vi "construct.vi"(8 "error in (no error)":errorcluster, 9 "configuration name":string, 10 "load config file?":bool=TRUE, 11 "StimulatorDL090824Gate in":refnum<class "StimulatorDL090824Gate.lvclass">) -> (0 "error out":errorcluster, 3 "StimulatorDL090824Gate out":refnum<class "StimulatorDL090824Gate.lvclass">)   [LabVIEW 2010, in "StimulatorDL090824Gate.lvclass"]
uses:
  StimulatorDL090824Gate.lvclass
  StimulatorDL090724Scaffold/StimulatorDL090724Scaffold/Stimulator090724Scaffold.lvclass
  StimulatorDL090824Gate.lvclass/StimulatorDL090824Gate.ctl
  common/classes/ErrorController/ErrorController/class_data.vi
  common/classes/ErrorController/ErrorController/ErrorController.lvclass
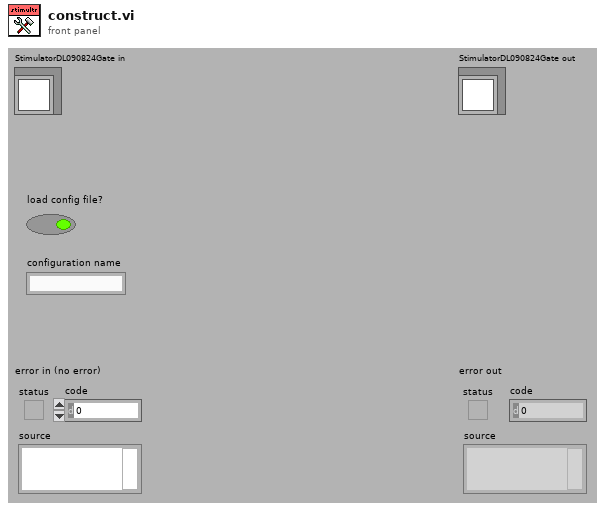
[diagram p1: front panel]
types:
  T1 = typedef "plugin_specification.ctl" = cluster{"class path":string, "configuration":string, "label":string, "settings name":string}
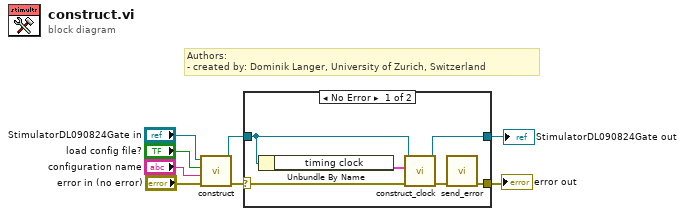
[diagram p0: block diagram]
diagram:
  # "Authors: \n- created by: Dominik Langer, University of Zurich, Switzerland"
  n1 = call-parent "construct.vi"("error in (no error)"="error in (no error)", "configuration name"="configuration name", "load config file?"="load config file?", "GenericPlugin in"="StimulatorDL090824Gate in") -> ("error out"=w4:errorcluster, "GenericPlugin out"=w3:refnum<class "StimulatorDL090824Gate.lvclass">)  [unwired: 6 in]
  n2 = case shown="No Error" w4 {
    selector: w4 -> [w14 w15]
    tunnel: w3 -> [w12 w16]
    tunnel: [w11 w16] -> w2
    tunnel: [w9 w15] -> w1
    frame No Error {
      n3 = Unbundle By Name(w12) -> ("timing clock"=w13:T1)
      n4 = call-dynamic "construct_clock.vi"("error in (no error)"=w14, "clock specification"=w13, "Stimulator090724Scaffold in"=w12) -> ("error out"=w10:errorcluster, "Stimulator090724Scaffold out"=w11:refnum<class "StimulatorDL090824Gate.lvclass">)  [unwired: 7 in]
      n5 = call "send_error.vi"("error in (no error)"=w10) -> ("error out"=w9:errorcluster)  [unwired: 10 in]
    }
    frame Error {
    }
  }
  "error out" <- w1
  "StimulatorDL090824Gate out" <- w2
